vi "Read Preloaded Configuration.vi"(11 "TransientConfiguration in":refnum<class "TransientConfiguration.lvclass">) -> (2 "Pre-Loaded Configuration":variant, 3 "TransientConfiguration out":refnum<class "TransientConfiguration.lvclass">)   [LabVIEW 2017, in "TransientConfiguration.lvclass"]
uses:
  TransientConfiguration.lvclass
  TransientConfiguration.lvclass/TransientConfiguration.ctl
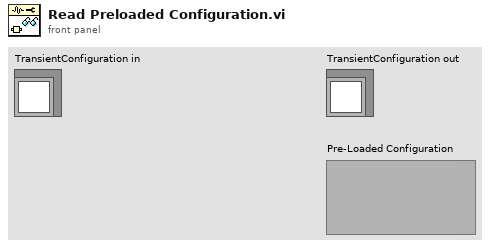
[diagram p1: front panel]
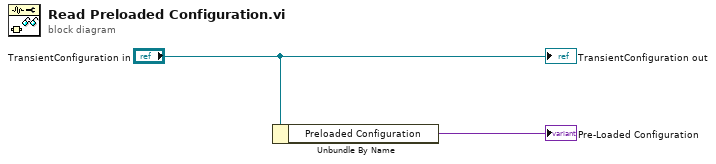
[diagram p0: block diagram]
diagram:
  n1 = Unbundle By Name("TransientConfiguration in") -> ("Preloaded Configuration"=→"Pre-Loaded Configuration":variant)
  "TransientConfiguration out" <- "TransientConfiguration in"
